vi "Pre Launch Init.vi"(11 "Chamber Controller in":refnum<class "Chamber Controller.lvclass">) -> (0 "error out":errorcluster, 3 "Chamber Controller out":refnum<class "Chamber Controller.lvclass">)   [LabVIEW 2020, in "Chamber Controller.lvlib" / "Chamber Controller.lvclass"]
doc: "(<B>Filename</B>: Actor Framework.lvlib:Actor.lvclass:Pre Launch Init.vi)\n\nDefines behavior that occurs after the Launch Nested Actor method is invoked but before the actor's Actor Core method begins running.\n\nBy default, this method does nothing. A descendant class may override it to define behavior."
uses:
  Chamber Controller.lvclass
  _Abstract Classes/Abstract Chamber/Abstract Chamber.lvclass
  Chamber Controller.lvclass/Chamber Controller.ctl
  <vilib>/MGI/Monitored Actor/Monitored Actor/Monitored Actor/Monitored Actor.lvclass
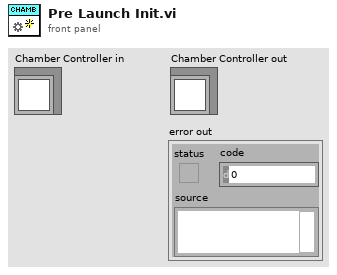
[diagram p1: front panel]
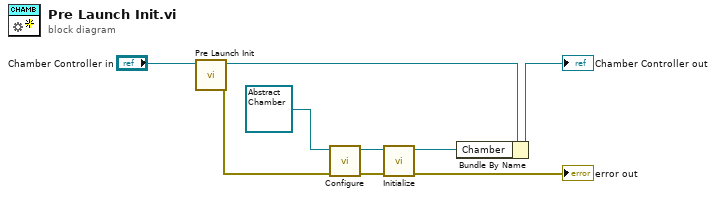
[diagram p0: block diagram]
diagram:
  n1 = call-parent "Pre Launch Init.vi"("Monitored Actor in"="Chamber Controller in") -> ("error out"=w1:errorcluster, "Monitored Actor out"=w8:refnum<class "Chamber Controller.lvclass">)  [unwired: 9 in]
  n2 = call-dynamic "Configure.vi"("error in (no error)"=w1, "Chamber in"=refnum<class "Abstract Chamber.lvclass"> refnum ("Chamber Controller.lvlib:Abstract Chamber.lvclass")) -> ("error out"=w5:errorcluster, "Chamber out"=w6:refnum<class "Abstract Chamber.lvclass">)  [unwired: 8 in]
  n3 = call-dynamic "Initialize.vi"("error in (no error)"=w5, "Chamber in"=w6) -> ("error out"=→"error out":errorcluster, "Chamber out"=w4:refnum<class "Abstract Chamber.lvclass">)  [unwired: 8 in]
  n4 = Bundle By Name(cluster=w8, "Chamber"=w4) -> (→"Chamber Controller out":refnum<class "Chamber Controller.lvclass">)
